vi "Get_fast_seq_info.vi"(1 "ConfigFilePath":path) -> (0 "Fast sequence parameters":T7 {"fastseq"."DAC"."DAC offset" min=-1 max=0.5; "fastseq"."DAC"."FastChanNum" max=15 step=1; "fastseq"."slot#" max=4095})   [LabVIEW 2013]
uses:
  sequence slot/slot-use.ctl
  sequence slot/triggers.ctl
  sequence slot/DAC.ctl
  sequence slot/DAC_fastseq-offset.ctl
  sequence slot/timing.ctl
  sequence slot/jump.ctl
  <vilib>/addons/h5labview2/file/H5Fmode.ctl
  <vilib>/addons/h5labview2/base/lib_path.vi
  <vilib>/addons/h5labview2/base/H5Equery.vi
  <vilib>/addons/h5labview2/base/hid_t.ctl
  <vilib>/addons/h5labview2/dataset/H5Dread.llb/H5Dread.xnode
  <vilib>/addons/h5labview2/attrib/H5Aread.llb/H5Aread.xnode
  <vilib>/addons/h5labview2/file/H5F.lvlib
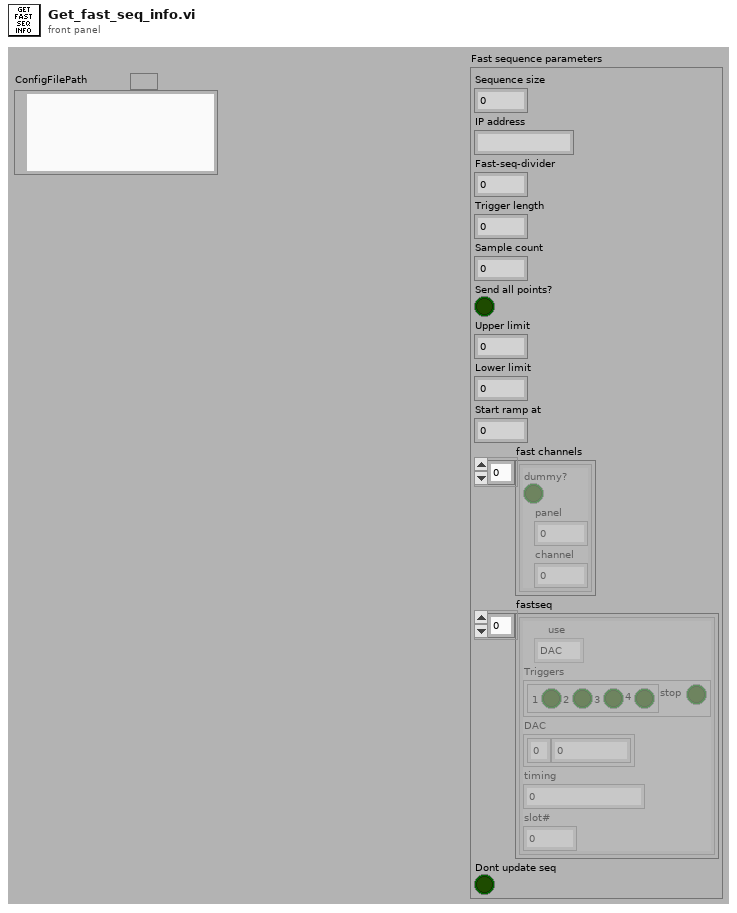
[diagram p1: front panel]
types:
  T1 = typedef "slot-use.ctl" = enum8{"DAC", "timing", "triggers", "jump"}
  T2 = typedef "triggers.ctl" = cluster{"triggers":cluster{"1":bool, "2":bool, "3":bool, "4":bool}, "stop":bool}
  T3 = typedef "DAC.ctl" = cluster{"FastChanNum":u8, "DAC offset":T4}
  T4 = typedef "DAC_fastseq-offset.ctl" = sgl
  T5 = typedef "timing.ctl" = sgl
  T6 = typedef "jump.ctl" = u16
  T7 = cluster{"Sequence size":u64, "IP address":string, "Fast-seq-divider":u64, "Trigger length":u64, "Sample count":u64, "Send all points?":bool, "Upper limit":dbl, "Lower limit":dbl, "Start ramp at":u64, "fast channels":cluster{"dummy?":bool, "panel":u8, "channel":u8}[], "fastseq":cluster{"use":T1, "Triggers":T2, "DAC":T3, "timing":T5, "slot#":T6}[], "Dont update seq":bool}
  T8 = cluster{"Sequence size":u64, "IP address":string, "Fast-seq-divider":u64, "Trigger length":u64, "Sample count":u64, "Send all points?":bool, "Upper limit":dbl, "Lower limit":dbl, "Start ramp at":u64, "fast channels":cluster{"dummy?":bool, "panel":u8, "channel":u8}[], "fastseq":cluster{"use":T1, "Triggers":T2, "DAC":T3, "timing":T5, "slot#":T6}[], "don't update seq":bool}
  T9 = typedef "H5F.lvlib/H5Fmode.ctl" = enum16{"read-only", "read-write", "overwrite", "create new", "open or create"}
  T10 = typedef "hid_t.ctl" = i32
  T11 = cluster{"dummy?":bool, "panel":u8, "channel":u8}[]
  T12 = cluster{"use":T1, "Triggers":T2, "DAC":T3, "timing":T5, "slot#":T6}[]
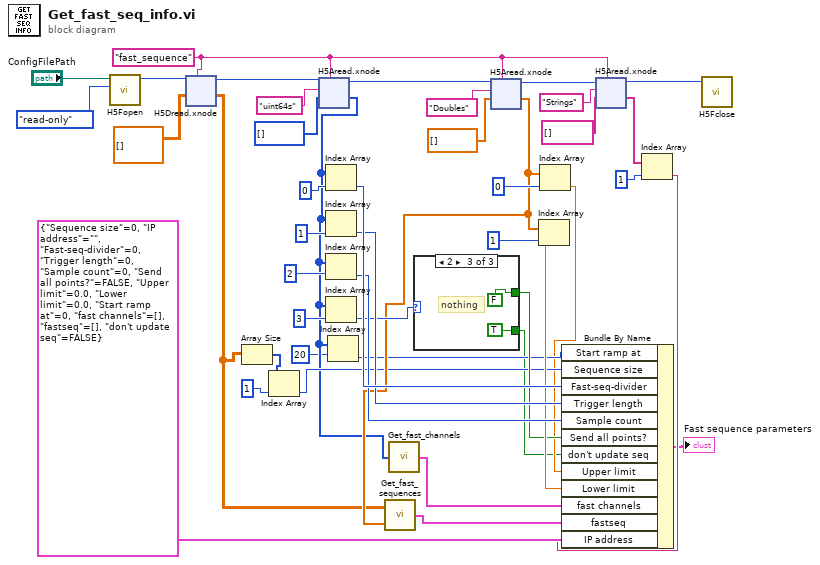
[diagram p0: block diagram]
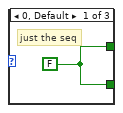
[diagram p2: hidden frame]
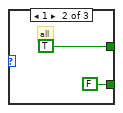
[diagram p3: hidden frame]
diagram:
  w17 = "fast_sequence"
  n1 = call <vilib>:"H5Fopen.vi"("mode (read-only)"=H5Fmode."read-only" ("mode"), "path"="ConfigFilePath") -> ("ref out"=w42:T10)  [unwired: 8 in, 1 out]
  n2 = xnode "H5Dread.xnode"("dataset name (this)"=w17, "default"=dbl[][] [], "ref in"=w42) -> ("data"=w10:dbl[][], "ref out"=w38:T10)  [unwired: 3 in, 2 out]
  n3 = Array Size(array=w10) -> (size(s)=w8:i32[])
  n4 = Index Array(array=w8, index=1) -> (element=w7:i32)
  n5 = xnode "H5Aread.xnode"("object name"=w17, "default"=u64[] [], "attrib name"="uint64s", "ref in"=w38) -> ("data"=w5:u64[], "ref out"=w35:T10)  [unwired: 2 in, 2 out]
  n6 = Index Array(array=w5, index=0) -> (element=w30:u64)
  n7 = Index Array(array=w5, index=1) -> (element=w29:u64)
  n8 = Index Array(array=w5, index=2) -> (element=w28:u64)
  n9 = Index Array(array=w5, index=3) -> (element=w24:u64)
  n10 = Index Array(array=w5, index=20) -> (element=w3:u64)
  n11 = call "Get_fast_channels.vi"("uint16s"=w5) -> ("Fast channels"=w22:T11)
  n12 = case shown="2" w24 {
    tunnel: [w45 TRUE FALSE] -> w23
    tunnel: [w45 FALSE TRUE] -> w1
    frame 0, Default {
      w45 = FALSE
      # "just the seq"
    }
    frame 1 {
      # "all"
    }
    frame 2 {
      # "nothing"
    }
  }
  n13 = xnode "H5Aread.xnode"("object name"=w17, "default"=dbl[] [], "attrib name"="Doubles", "ref in"=w35) -> ("data"=w21:dbl[], "ref out"=w19:T10)  [unwired: 2 in, 2 out]
  n14 = call "Get_fast_sequences.vi"("Doubles"=w21, "Array"=w10) -> ("Fast sequence"=w20:T12)
  n15 = Index Array(array=w21, index=1) -> (element=w25:dbl)
  n16 = Index Array(array=w21, index=0) -> (element=w2:dbl)
  n17 = xnode "H5Aread.xnode"("object name"=w17, "default"=string[] [], "attrib name"="Strings", "ref in"=w19) -> ("data"=w14:string[], "ref out"=w18:T10)  [unwired: 2 in, 2 out]
  n18 = Index Array(array=w14, index=1) -> (element=w11:string)
  n19 = Bundle By Name(cluster=T8 {"Sequence size"=0, "IP address"="", "Fast-seq-divider"=0, "Trigger length"=0, "Sample count"=0, "Send all points?"=FALSE, "Upper limit"=0.0, "Lower limit"=0.0, "Start ramp at"=0, "fast channels"=[], "fastseq"=[], "don't update seq"=FALSE} ("Fast sequence parameters 2"), "Start ramp at"=w3, "Sequence size"=w7, "Fast-seq-divider"=w30, "Trigger length"=w29, "Sample count"=w28, "Send all points?"=w23, "don't update seq"=w1, "Upper limit"=w2, "Lower limit"=w25, "fast channels"=w22, "fastseq"=w20, "IP address"=w11) -> (→"Fast sequence parameters":T8)
  n20 = call <vilib>:"H5Fclose.vi"("ref"=w18) -> ()  [unwired: 10 in, 1 out]
